vi "QVA_DeleteVariantAttributes.vi"(0 "QueueIn":refnum<queue>, 1 "Name":string[](array[string]), 5 "ErrorIn":errorcluster, 9 "Timeout":i32=-1) -> (14 "QueueOut":refnum<queue>, 16 "Timeout":bool, 17 "FoundAndRemoved":bool, 19 "ErrorOut":errorcluster)   [LabVIEW 2016]
doc: "Löscht mehrere Variant Attributes aus dem QVA\n\nsige / 3.12.13"
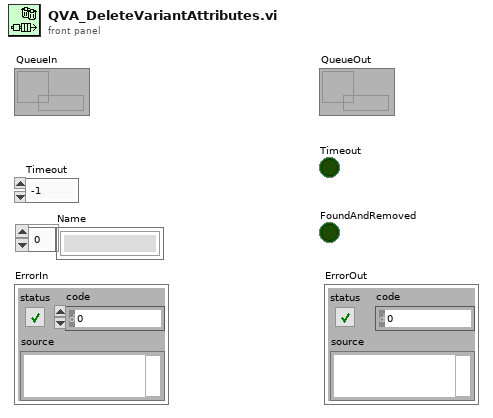
[diagram p1: front panel]
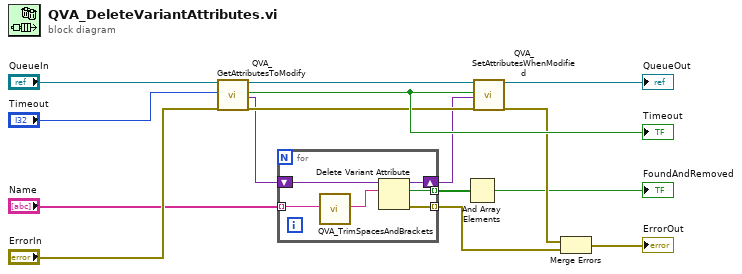
[diagram p0: block diagram]
diagram:
  n1 = call "QVA_GetAttributesToModify.vi"("QueueIn"="QueueIn", "Timeout"="Timeout", "ErrorIn"="ErrorIn") -> ("QueueOut"=w8:refnum<queue>, "Timeout"=w12:bool, "VariantData"=w5:variant, "ErrorOut"=w6:errorcluster)  [unwired: 13 in]
  "Timeout" <- w12
  n2 = for {
    tunnel: [w21] -> w9 mode=indexing
    tunnel: [w18] -> w3 mode=indexing
    tunnel: "Name" -> [w17] mode=indexing
    shift-right: [w19] -> w4
    shift-left: w5 -> [w20]
    n3 = call "QVA_TrimSpacesAndBrackets.vi"("String"=w17) -> ("TrimmedString"=w16:string)  [unwired: 18 in]
    n4 = Delete Variant Attribute(6:w16, 7:w20) -> (0:w18:errorcluster, 2:w21:bool, 3:w19:variant)  [unwired: 1 in]
  }
  n5 = And Array Elements(Boolean array=w9) -> (logical AND=→"FoundAndRemoved":bool)
  n6 = call "QVA_SetAttributesWhenModified.vi"("QueueIn"=w8, "SkipAfterTimeout"=w12, "VariantData"=w4, "ErrorIn"=w6) -> ("QueueOut"=→"QueueOut":refnum<queue>, "ErrorOut"=w7:errorcluster)  [unwired: 14 in]
  n7 = Merge Errors(w7, w3) -> (→"ErrorOut":errorcluster)
